vi "SerialPort.Read.vi"(8 "error in (no error)":errorcluster, 11 "SerialPort in":refnum<class "SerialPort.lvclass">) -> (0 "error out":errorcluster, 1 "Data":string, 2 "State":T1, 3 "SerialPort out":refnum<class "SerialPort.lvclass">)   [LabVIEW 2018, in "SerialPort.lvclass"]
uses:
  SerialPort.lvclass
  Controls/SerialPort.Status Enum.ctl
  SerialPort.lvclass/SerialPort.ctl
  Utils/Errors/Error.Error Code List.ctl
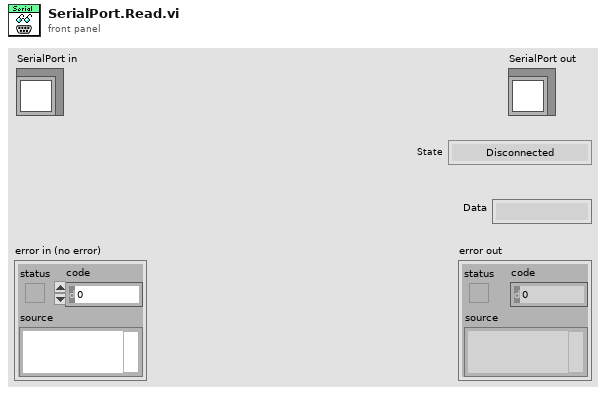
[diagram p1: front panel]
types:
  T1 = typedef "SerialPort.Status Enum.ctl" = enum16{"Disconnected", "Connecting", "Connected"}
  T2 = typedef "Error.Error Code List.ctl" = i32
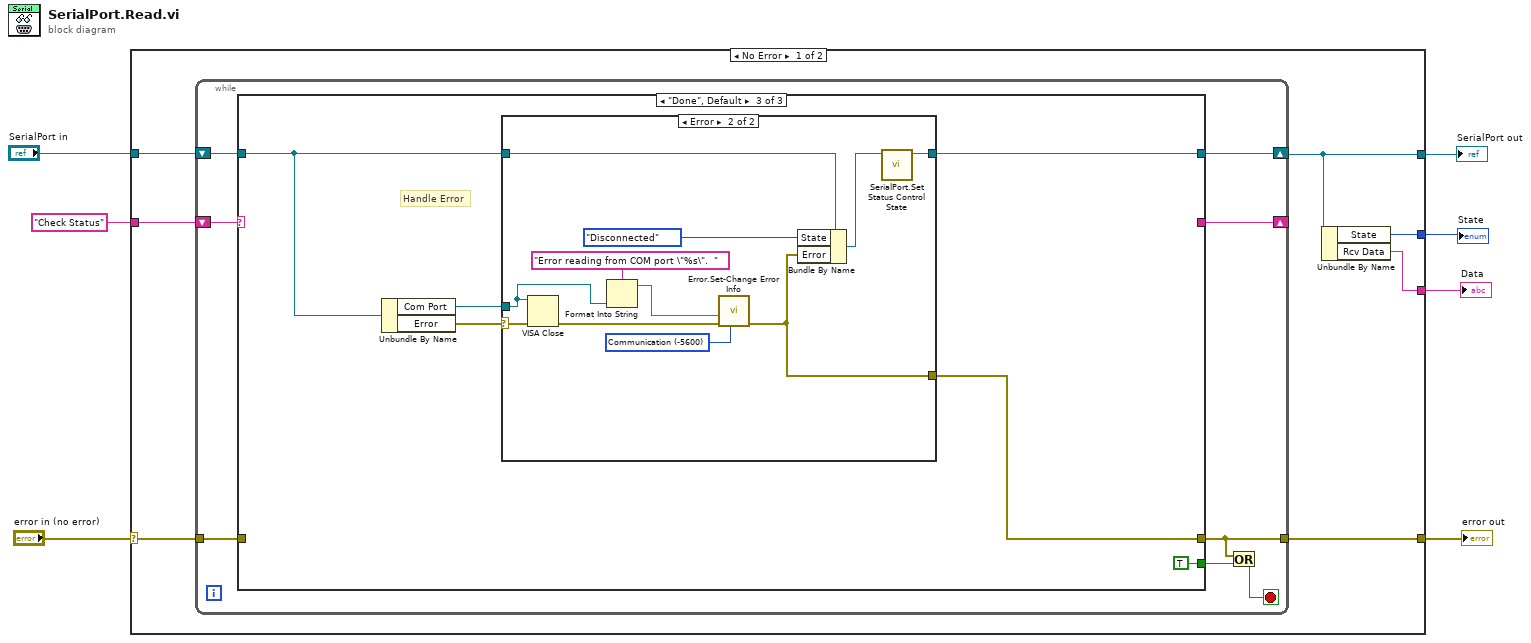
[diagram p0: block diagram]
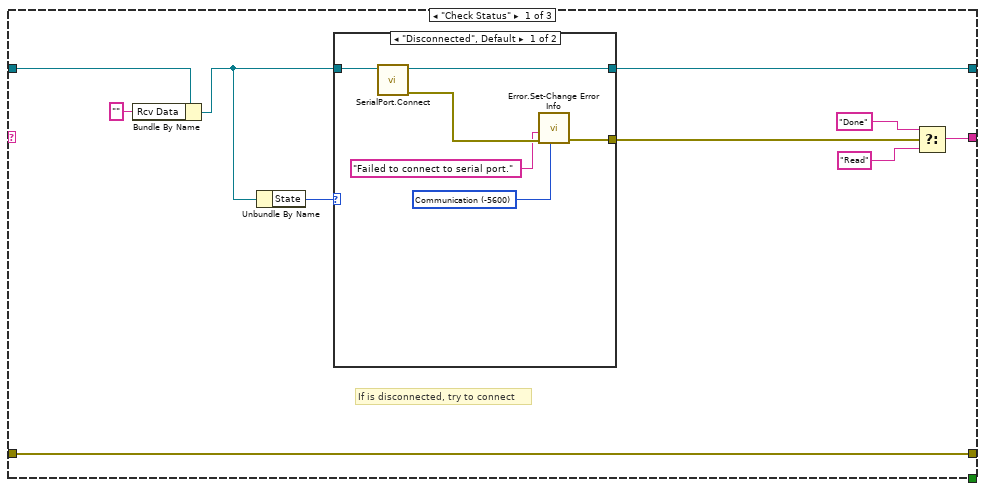
[diagram p2: hidden frame]
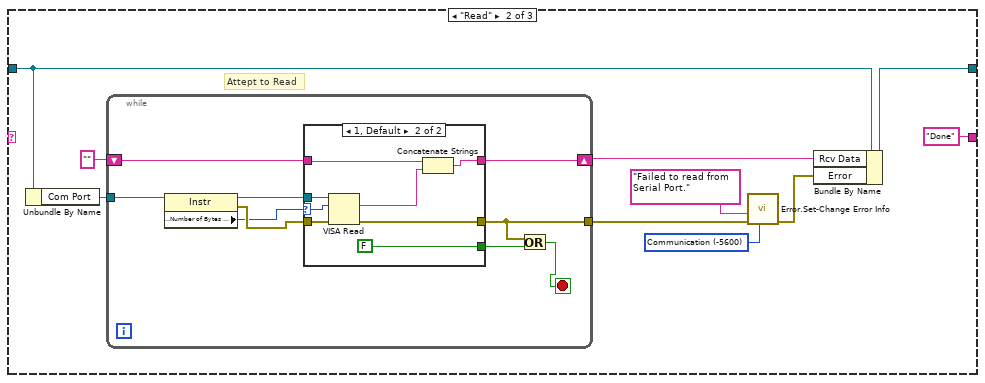
[diagram p4: hidden frame]
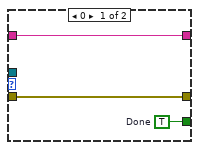
[diagram p5: hidden frame]
diagram:
  n1 = case shown="No Error" "error in (no error)" {
    selector: "error in (no error)" -> [w8 w89]
    tunnel: [w12 w89] -> w6
    tunnel: [w11 w88] -> w4
    tunnel: "SerialPort in" -> [w14 w88]
    tunnel: "Check Status" -> [w13 _]
    tunnel: [w9 _] -> w2
    tunnel: [w10 _] -> w1
    frame No Error {
      n2 = while {
        shift-right: [w20] -> w11
        shift-left: w14 -> [w21]
        shift-right: [w19] -> _
        shift-left: w13 -> [w22]
        tunnel: [w18] -> w12
        tunnel: w8 -> [w15]
        stop <- w16 stop-if-true
        n3 = case shown="\"Done\", Default" w22 {
          tunnel: w21 -> [w26 w46 w74]
          tunnel: [w31 w44 w70] -> w20
          tunnel: [w30 "Done" _] -> w19
          tunnel: [w23 _ w72] -> w18
          tunnel: [_ _ TRUE] -> w17
          tunnel: w15 -> [w23 _ _]
          frame "Check Status" {
            # "If is disconnected, try to connect"
            n4 = Bundle By Name(cluster=w26, "Rcv Data"="") -> (w25:refnum<class "SerialPort.lvclass">)
            n5 = Unbundle By Name(w25) -> ("State"=w32:T1)
            n6 = case shown="\"Disconnected\", Default" w32 {
              tunnel: w25 -> [w38 w39]
              tunnel: [w37 w39] -> w31
              tunnel: [w36 _] -> w29
              frame "Disconnected", Default {
                w35 = T2 -5600 items=["No Error"=0, "Abort"=-2, "Misc"=-5000, "Fixture Error"=-5100, "File IO - General"=-5200, "FIle IO - Config Error"=-5201, "Instrument - General"=-5300, "Instrument - Serial Com"=-5301, "Instrument - Camera"=-5302, "Instrument - PS"=-5303, "Instrument - Oscilloscope"=-5304, "Instrument - Function Gen"=-5305, "Instrument - Load"=-5306, "Instrument - Meter"=-5307, "Instrument - Power Control"=-5308, "Instrument - Motion"=-5309, "Instrument - RF"=-5310, "System Exe"=-5400, "Image Processing"=-5500, "Communication"=-5600, "Script - Syntax Error"=-6000, "Script - Invalid Name or Param"=-6100, "Script - Timeout"=-6200, "Invalid Data"=-6300] ("Std Code")
                n7 = call "SerialPort.Connect.vi"("SerialPort in"=w38) -> ("error out"=w34:errorcluster, "SerialPort out"=w37:refnum<class "SerialPort.lvclass">)  [unwired: 8 in, 1 out]
                n8 = call "Error.Set-Change Error Info.vi"("Std Code"=w35, "error in"=w34, "Description"="Failed to connect to serial port.") -> ("error out"=w36:errorcluster)  [unwired: 8 in]
              }
              frame "Connected" {
              }
            }
            n9 = Select(t="Done", s=w29, f="Read") -> (s? t:f=w30:string)
          }
          frame "Read" {
            w41 = T2 -5600 items=["No Error"=0, "Abort"=-2, "Misc"=-5000, "Fixture Error"=-5100, "File IO - General"=-5200, "FIle IO - Config Error"=-5201, "Instrument - General"=-5300, "Instrument - Serial Com"=-5301, "Instrument - Camera"=-5302, "Instrument - PS"=-5303, "Instrument - Oscilloscope"=-5304, "Instrument - Function Gen"=-5305, "Instrument - Load"=-5306, "Instrument - Meter"=-5307, "Instrument - Power Control"=-5308, "Instrument - Motion"=-5309, "Instrument - RF"=-5310, "System Exe"=-5400, "Image Processing"=-5500, "Communication"=-5600, "Script - Syntax Error"=-6000, "Script - Invalid Name or Param"=-6100, "Script - Timeout"=-6200, "Invalid Data"=-6300] ("Std Code")
            # "Attept to Read"
            n10 = Unbundle By Name(w46) -> ("Com Port"=w49:refnum<visa-resource-name>)
            n11 = while {
              tunnel: w49 -> [w57]
              tunnel: [w52] -> w42
              shift-right: [w50] -> w45
              shift-left: "" -> [w51]
              stop <- w53 stop-if-true
              n12 = property class="Instr"(reference=w57) -> (reference out=w58:refnum<visa-resource-name>, error out=w56:errorcluster, "Serial Settings:Number of Bytes at Serial Port"=w55:u32)  [unwired: 1 in]
              n13 = case shown="1, Default" w55 {
                selector: w55 -> [_ w67]
                tunnel: w58 -> [_ w69]
                tunnel: w56 -> [w61 w68]
                tunnel: [w61 w66] -> w52
                tunnel: [w60 FALSE] -> w54
                tunnel: w51 -> [w59 w63]
                tunnel: [w59 w64] -> w50
                frame 0 {
                  w60 = TRUE  # Done
                }
                frame 1, Default {
                  n14 = VISA Read(VISA resource name=w69, byte count=w67, error in (no error)=w68) -> (read buffer=w62:string, error out=w66:errorcluster)  [unwired: 2 out]
                  n15 = Concatenate Strings(w63, w62) -> (w64:string)
                }
              }
              n16 = Or(x=w52, y=w54) -> (x .or. y?=w53:bool)
            }
            n17 = call "Error.Set-Change Error Info.vi"("Std Code"=w41, "error in"=w42, "Description"="Failed to read from Serial Port.") -> ("error out"=w43:errorcluster)  [unwired: 8 in]
            n18 = Bundle By Name(cluster=w46, "Rcv Data"=w45, "Error"=w43) -> (w44:refnum<class "SerialPort.lvclass">)
          }
          frame "Done", Default {
            # "Handle Error"
            n19 = Unbundle By Name(w74) -> ("Com Port"=w73:refnum<visa-resource-name>, "Error"=w75:errorcluster)
            n20 = case shown="Error" w75 {
              selector: w75 -> [w77 w81]
              tunnel: w74 -> [w76 w85]
              tunnel: [w76 w83] -> w70
              tunnel: w73 -> [_ w84]
              tunnel: [w77 w79] -> w72
              frame No Error {
              }
              frame Error {
                w78 = T2 -5600 items=["No Error"=0, "Abort"=-2, "Misc"=-5000, "Fixture Error"=-5100, "File IO - General"=-5200, "FIle IO - Config Error"=-5201, "Instrument - General"=-5300, "Instrument - Serial Com"=-5301, "Instrument - Camera"=-5302, "Instrument - PS"=-5303, "Instrument - Oscilloscope"=-5304, "Instrument - Function Gen"=-5305, "Instrument - Load"=-5306, "Instrument - Meter"=-5307, "Instrument - Power Control"=-5308, "Instrument - Motion"=-5309, "Instrument - RF"=-5310, "System Exe"=-5400, "Image Processing"=-5500, "Communication"=-5600, "Script - Syntax Error"=-6000, "Script - Invalid Name or Param"=-6100, "Script - Timeout"=-6200, "Invalid Data"=-6300] ("Std Code")
                n21 = VISA Close(VISA resource name=w84) -> ()  [unwired: 1 in, 1 out]
                n22 = Format Into String(format string="Error reading from COM port \"%s\".  ", w84) -> (resulting string=w80:string)  [unwired: 2 in, 1 out]
                n23 = call "Error.Set-Change Error Info.vi"("Std Code"=w78, "error in"=w81, "Description"=w80) -> ("error out"=w79:errorcluster)  [unwired: 8 in]
                n24 = Bundle By Name(cluster=w85, "State"=SerialPort.Status_Enum."Disconnected", "Error"=w79) -> (w82:refnum<class "SerialPort.lvclass">)
                n25 = call "SerialPort.Set Status Control State.vi"("SerialPort in"=w82) -> ("SerialPort out"=w83:refnum<class "SerialPort.lvclass">)  [unwired: 9 in, 1 out]
              }
            }
          }
        }
        n26 = Or(x=w18, y=w17) -> (x .or. y?=w16:bool)
      }
      n27 = Unbundle By Name(w11) -> ("State"=w10:T1, "Rcv Data"=w9:string)
    }
    frame Error {
    }
  }
  "error out" <- w6
  "SerialPort out" <- w4
  "Data" <- w2
  "State" <- w1
